vi "Set Glue Reservoir Vacuum.vi"(8 "error in (no error)":errorcluster, 9 "On/Off":bool, 11 "Gantry Class in":refnum<class "Gantry Class.lvclass">) -> (0 "error out":errorcluster, 3 "Gantry Class out":refnum<class "Gantry Class.lvclass">)   [LabVIEW 2011, in "Gantry Class.lvclass"]
uses:
  Gantry Class.lvclass
  WorkTable Class/WorkTable Class.lvclass
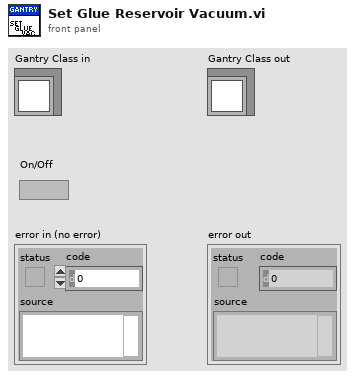
[diagram p1: front panel]
types:
  T1 = typedef "Worktable_Glue Reservoir.ctl" = cluster{"Glue Reservoir Slots":cluster{"Reservoir State":enum16{"Empty", "Full", "Used"}, "Center":refnum<class "Vec3d Class.lvclass">}[], "Vacuum Channel":i32}
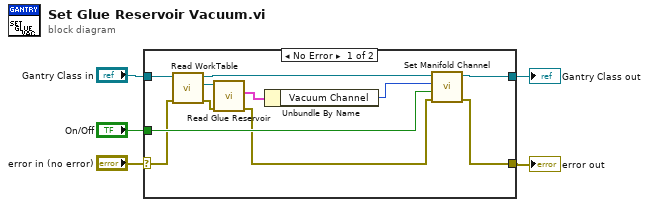
[diagram p0: block diagram]
diagram:
  n1 = case shown="No Error" "error in (no error)" {
    selector: "error in (no error)" -> [w7 w18]
    tunnel: [w12 w18] -> w2
    tunnel: [w13 w17] -> w1
    tunnel: "Gantry Class in" -> [w16 w17]
    tunnel: "On/Off" -> [w15 _]
    frame No Error {
      n2 = call-dynamic "Read WorkTable.vi"("error in"=w7, "Gantry Class in"=w16) -> ("error out"=w8:errorcluster, "WorkTable Class.lvclass"=w11:refnum<class "WorkTable Class.lvclass">, "Gantry Class out"=w14:refnum<class "Gantry Class.lvclass">)  [unwired: 7 in]
      n3 = call-dynamic "Read Glue Reservoir.vi"("error in (no error)"=w8, "WorkTable Class in"=w11) -> ("error out"=w6:errorcluster, "Glue Reservoir"=w10:T1)  [unwired: 7 in, 1 out]
      n4 = Unbundle By Name(w10) -> ("Vacuum Channel"=w9:i32)
      n5 = call-dynamic "Set Manifold Channel.vi"("error in"=w6, "On/Off"=w15, "Manifold Channel"=w9, "Gantry in"=w14) -> ("error out"=w12:errorcluster, "Gantry out"=w13:refnum<class "Gantry Class.lvclass">)  [unwired: 6 in]
    }
    frame Error {
    }
  }
  "error out" <- w2
  "Gantry Class out" <- w1
